vi "Write Data.vi"(8 "error in (no error)":errorcluster, 9 "Publication Time":timestamp, 10 "Value":variant, 11 "ActorDataBinding in":refnum<class "ActorDataBinding.lvclass">) -> (0 "error out":errorcluster, 3 "ActorDataBinding out":refnum<class "ActorDataBinding.lvclass">)   [LabVIEW 2017, in "IObserver.lvlib" / "ActorDataBinding.lvclass"]
doc: "<License>\nCopyright © 2017 Composed Systems, LLC | All rights reserved\nwww.composed.io\n\nAuthor: Ethan Stern <ethan.stern@composed.io>\n\nThis software is provided \"AS IS\" WITHOUT WARRANTIES, either express or implied, AND IS FOR EDUCATIONAL PURPOSES ONLY.\n</License>"
uses:
  ActorDataBinding.lvclass
  ActorDataBinding.lvclass/ActorDataBinding.ctl
  IObserver Messages/Observe Data Msg/Observe Data Msg.lvclass
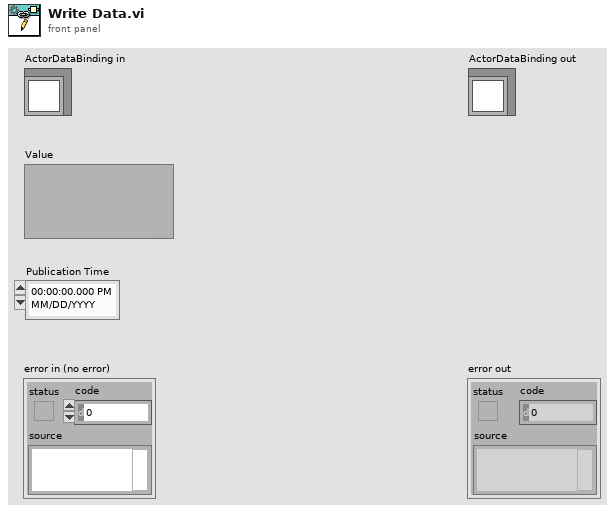
[diagram p1: front panel]
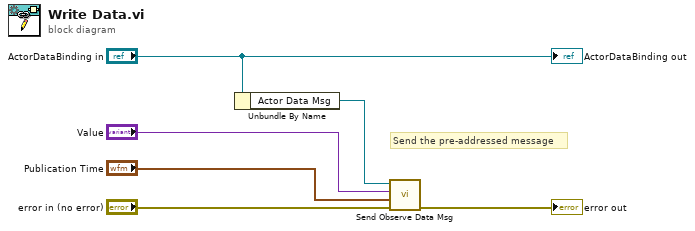
[diagram p0: block diagram]
diagram:
  # "Send the pre-addressed message"
  n1 = Unbundle By Name("ActorDataBinding in") -> ("Actor Data Msg"=w5:refnum<class "Observe Data Msg.lvclass">)
  n2 = call "Send Observe Data Msg.vi"("error in (no error)"="error in (no error)", "Publication Time (Use Current Time)"="Publication Time", "Value"="Value", "Actor Data Msg In"=w5) -> ("error out"=→"error out":errorcluster)  [unwired: 7 in]
  "ActorDataBinding out" <- "ActorDataBinding in"
